vi "Frame Process.vi"(8 "error in (no error)":errorcluster, 10 "Video Frame In":refnum<class "Video Frame.lvclass">, 11 "EdgeDetectionProcessor in":refnum<class "EdgeDetectionProcessor.lvclass">) -> (0 "error out":errorcluster, 3 "EdgeDetectionProcessor out":refnum<class "EdgeDetectionProcessor.lvclass">)   [LabVIEW 2018, in "EdgeDetectionProcessor.lvclass"]
uses:
  EdgeDetectionProcessor.lvclass
  C:/Program Files/National Instruments/LabVIEW 2018/user.lib/Aaron/File IO/Video/Video File/Video File.lvclass
  C:/Program Files/National Instruments/LabVIEW 2018/user.lib/Aaron/File IO/Video/Video Processor/Video Processor.lvclass
  <userlib>/Aaron/File IO/Video/Frames/Video Frame/Video Frame.lvclass
  <userlib>/Aaron/File IO/Video/Video Processor/Video Processor.lvclass
  <userlib>/Aaron/File IO/Video/Video File/Video File.lvclass
  <vilib>/vision/NI_Vision_Development_Module.lvlib
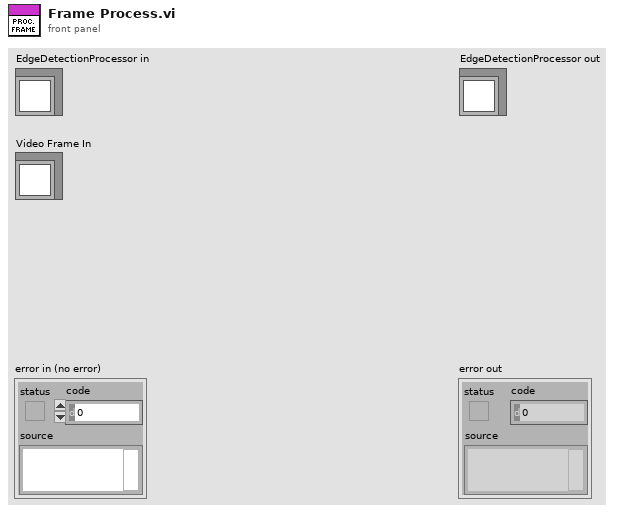
[diagram p1: front panel]
types:
  T1 = typedef "IMAQ Image.ctl" = refnum<image>
  T2 = cluster{"Global Rectangle":i32[], "Contours":cluster{"Contour Type":u32, "ROI Type":u32, "Points":i32[]}[]}
  T3 = typedef "IMAQ Curve Parameters.ctl" = cluster{"Extraction Mode":u32, "Edge Threshold":i32, "Edge Filter Size":u32, "Min Length":i32, "Row Search Step Size":i32, "Col Search Step Size":i32, "Max Endpoint Gap":i32, "Closed":bool, "Subpixel":bool}
  T4 = typedef "IMAQ ExtractCurvesCurve.ctl" = cluster{"Points":cluster{"X":dbl, "Y":dbl}[], "Closed?":bool, "Curve Length":dbl, "Min Edge Strength":dbl, "Max Edge Strength":dbl, "Average Edge Strength":dbl}
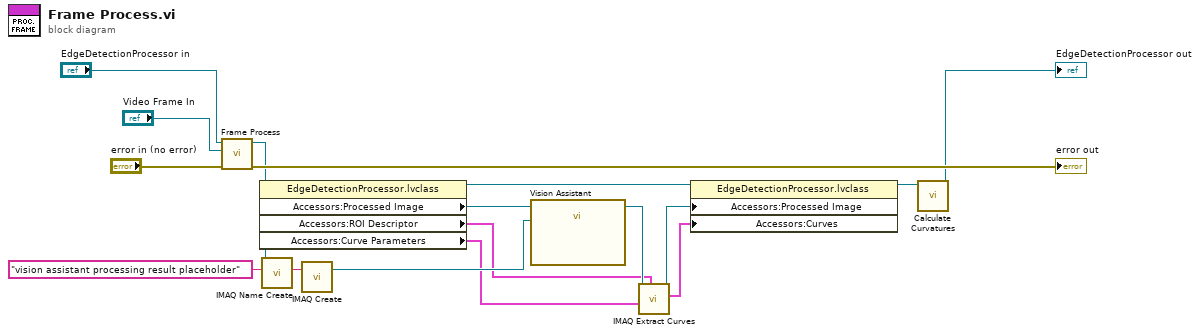
[diagram p0: block diagram]
diagram:
  n1 = call-parent "Frame Process.vi"("error in (no error)"="error in (no error)", "Video Frame In"="Video Frame In", "Video Processor in"="EdgeDetectionProcessor in") -> ("error out"=→"error out":errorcluster, "Video Processor out"=w11:refnum<class "EdgeDetectionProcessor.lvclass">)  [unwired: 7 in]
  n2 = property class="EdgeDetectionProcessor.lvclass"(reference=w11) -> (reference out=w12:refnum<class "EdgeDetectionProcessor.lvclass">, "Accessors:Processed Image"=w13:T1, "Accessors:ROI Descriptor"=w6:T2, "Accessors:Curve Parameters"=w3:T3)  [unwired: 1 in, 1 out]
  n3 = call <userlib>:"IMAQ Name Create.vi"("Name (\"\")"="vision assistant processing result placeholder" ("Name (\"\")"), "Video File in"=w11) -> ("Name Out"=w9:string)  [unwired: 7 in, 2 out]
  n4 = call "IMAQ Create"("Image Name"=w9) -> ("New Image"=w8:T1)  [unwired: 4 in, 1 out]
  n5 = call "Vision Assistant"("Image In"=w13, "Image Dst"=w8) -> ("Image Out"=w7:T1)  [unwired: 24 in, 1 out]
  n6 = call "IMAQ Extract Curves"("ROI Descriptor"=w6, "Curve Parameters"=w3, "Image"=w7) -> ("Curves"=w4:T4[], "Image (dup)"=w5:T1)  [unwired: 6 in, 1 out]
  n7 = property class="EdgeDetectionProcessor.lvclass"(reference=w12, "Accessors:Processed Image"=w5, "Accessors:Curves"=w4) -> (reference out=w2:refnum<class "EdgeDetectionProcessor.lvclass">)  [unwired: 1 in, 1 out]
  n8 = call-dynamic "Calculate Curvatures.vi"("EdgeDetectionProcessor in"=w2) -> ("EdgeDetectionProcessor out"=→"EdgeDetectionProcessor out":refnum<class "EdgeDetectionProcessor.lvclass">)  [unwired: 9 in, 1 out]
